vi "GetDescription.vi"(8 "error in (no error)":errorcluster caption="错误输入（无错误）", 11 "Beverage 输入":refnum<class "Beverage.lvclass">) -> (0 "error out":errorcluster caption="错误输出", 2 "Description":string, 3 "Beverage 输出":refnum<class "Beverage.lvclass">)   [LabVIEW 2016, in "Beverage.lvclass"]
uses:
  Beverage.lvclass
  Beverage.lvclass/Beverage.ctl
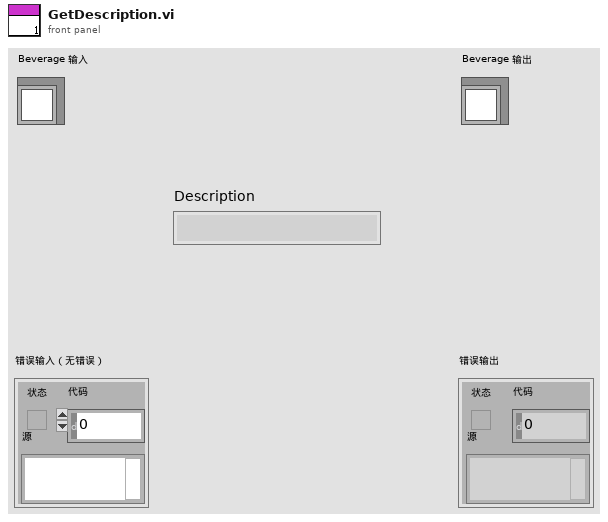
[diagram p1: front panel]
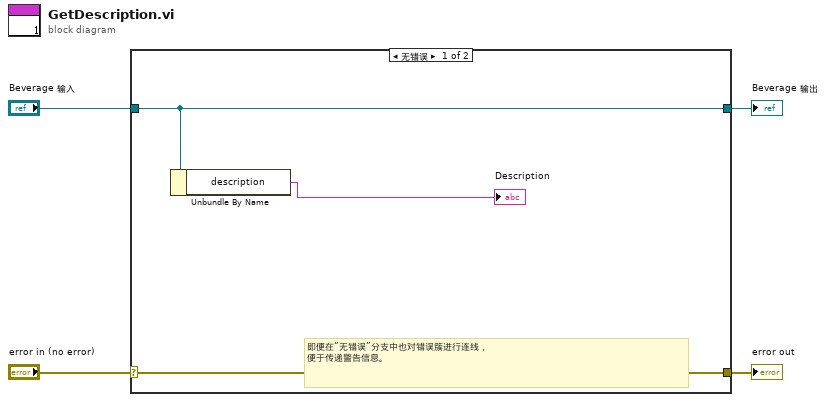
[diagram p0: block diagram]
diagram:
  n1 = case shown="无错误" "error in (no error)" {
    selector: "error in (no error)" -> [w7 w9]
    tunnel: [w7 w9] -> w3
    tunnel: [w6 w8] -> w1
    tunnel: "Beverage 输入" -> [w6 w8]
    frame No Error {
      # "即便在“无错误”分支中也对错误簇进行连线，\n便于传递警告信息。"
      n2 = Unbundle By Name(w6) -> ("description"=→"Description":string)
    }
    frame Error {
    }
  }
  "error out" <- w3
  "Beverage 输出" <- w1
